vi "file2DF2T.vi"(6 "Reset":bool, 9 "file path (use dialog)":path=path "c:/bob.dat", 11 "signal in":dbl) -> (3 "signal out":dbl)   [LabVIEW 2010, in "kevLib2010.lvlib"]
uses:
  kevLib2010.lvlib
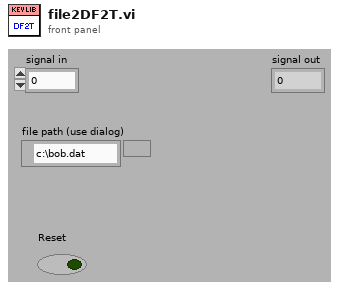
[diagram p1: front panel]
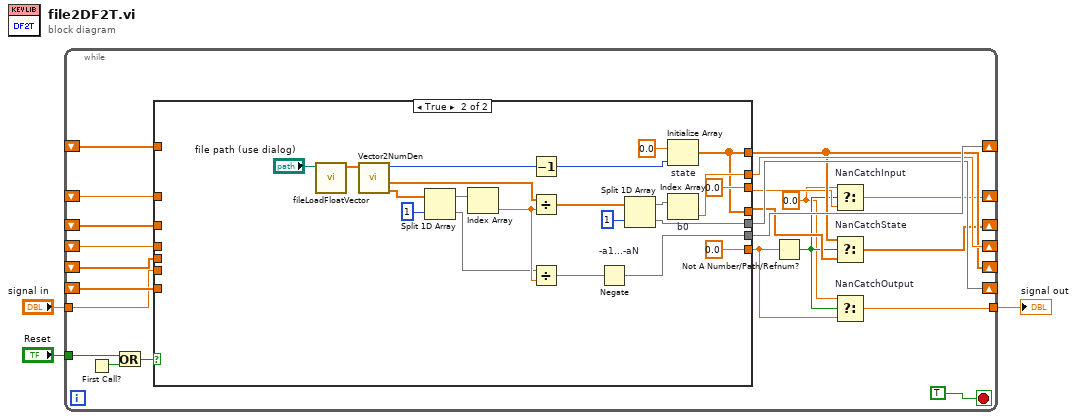
[diagram p0: block diagram]
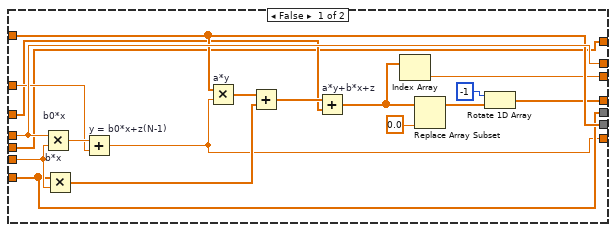
[diagram p2: hidden frame]
diagram:
  n1 = while {
    shift-right: [w13] -> _
    shift-left: _ -> [w19]
    shift-right: [w23] -> _
    shift-left: _ -> [w22]
    shift-right: [w24] -> _
    shift-left: _ -> [w21]
    shift-right: [w25] -> _
    shift-left: _ -> [w20]
    tunnel: "signal in" -> [w18]
    shift-right: [w11] -> _
    shift-left: _ -> [w17]
    tunnel: [w7] -> w2
    shift-right: [w15] -> _
    shift-left: _ -> [w16]
    tunnel: "Reset" -> [w4]
    stop <- TRUE stop-if-true
    w9 = 0.0 ("t")
    n2 = First Call?() -> (First Call?: T/F=w6:bool)
    n3 = Or(x=w4, y=w6) -> (x .or. y?=w5:bool)
    n4 = case shown="True" w5 {
      tunnel: [w44 w57] -> w23
      tunnel: [w39 w56] -> w24
      tunnel: [w41 w55] -> w25
      tunnel: [w28 w50] -> w14
      tunnel: w22 -> [w44 _]
      tunnel: w21 -> [w39 _]
      tunnel: w20 -> [w41 _]
      tunnel: w19 -> [w35 _]
      tunnel: w18 -> [w40 _]
      tunnel: w17 -> [w42 _]
      tunnel: [w34 0.0 ("Data Type (DBL)")] -> w12
      tunnel: [w33 0.0] -> w8
      tunnel: [w27 w50] -> w15
      tunnel: w16 -> [w27 _]
      frame False {
        n5 = Multiply "b0*x"(x=w44, y=w40) -> (x*y=w43:dbl)
        n6 = Multiply "b*x"(x=w39, y=w40) -> (x*y=w38:dbl[])
        n7 = Add "y = b0*x+z(N-1)"(x=w43, y=w42) -> (x+y=w33:dbl)
        n8 = Multiply "a*y"(x=w41, y=w33) -> (x*y=w37:dbl[])
        n9 = Add(x=w37, y=w38) -> (x+y=w36:dbl[])
        n10 = Add "a*y+b*x+z"(x=w36, y=w35) -> (x+y=w32:dbl[])
        n11 = Index Array(array=w32) -> (element=w34:dbl)  [unwired: 1 in]
        n12 = Replace Array Subset(array=w32, new element=0.0 ("new element/subarray")) -> (w30:dbl[])  [unwired: 1 in]
        n13 = Rotate 1D Array(1:w30, 2:-1 ("n")) -> (0:w28:dbl[])
      }
      frame True {
        n14 = call "fileLoadFloatVector.vi"("File Path"="file path (use dialog)") -> ("Float Vector"=w48:dbl[])  [unwired: 9 in, 1 out]
        n15 = call "Vector2NumDen.vi"("Filter Vector"=w48) -> ("Denominator"=w45:dbl[], "Numerator"=w46:dbl[], "FilterLength"=w47:i32)  [unwired: 8 in]
        n16 = Split 1D Array(array=w45, index=1) -> (first subarray=w63:dbl[], second subarray=w60:dbl[])
        n17 = Index Array(array=w63) -> (element=w62:dbl)  [unwired: 1 in]
        n18 = Decrement(x=w47) -> (x-1=w54:i32)
        n19 = Divide(x=w46, y=w62) -> (x/y=w61:dbl[])
        n20 = Divide(x=w60, y=w62) -> (x/y=w58:dbl[])
        n21 = Negate "-a1...-aN"(x=w58) -> (-x=w55:dbl[])
        n22 = Split 1D Array(array=w61, index=1) -> (first subarray=w59:dbl[], second subarray=w56:dbl[])
        n23 = Initialize Array "state"(0.0 ("element"), w54) -> (w50:dbl[])
        n24 = Index Array "b0"(array=w59) -> (element=w57:dbl)  [unwired: 1 in]
      }
    }
    n25 = Not A Number/Path/Refnum?(number/path/refnum=w8) -> (NaN/Path/Refnum?=w10:bool)
    n26 = Select "NanCatchInput"(t=w9, s=w10, f=w12) -> (s? t:f=w11:dbl)
    n27 = Select "NanCatchState"(t=w15, s=w10, f=w14) -> (s? t:f=w13:dbl[])
    n28 = Select "NanCatchOutput"(t=w9, s=w10, f=w8) -> (s? t:f=w7:dbl)
  }
  "signal out" <- w2
